vi "Modify Data format to R2 - 複製.vi"(8 "modified error":errorcluster, 10 "original error":errorcluster) -> ()   [LabVIEW 2023]
uses:
  <vilib>/Utility/error.llb/DialogType.ctl
panel:
  in  "Current set number in one current mode":i32=48
  in  "Scan number":i32=10
  out "element":string[](array[string])
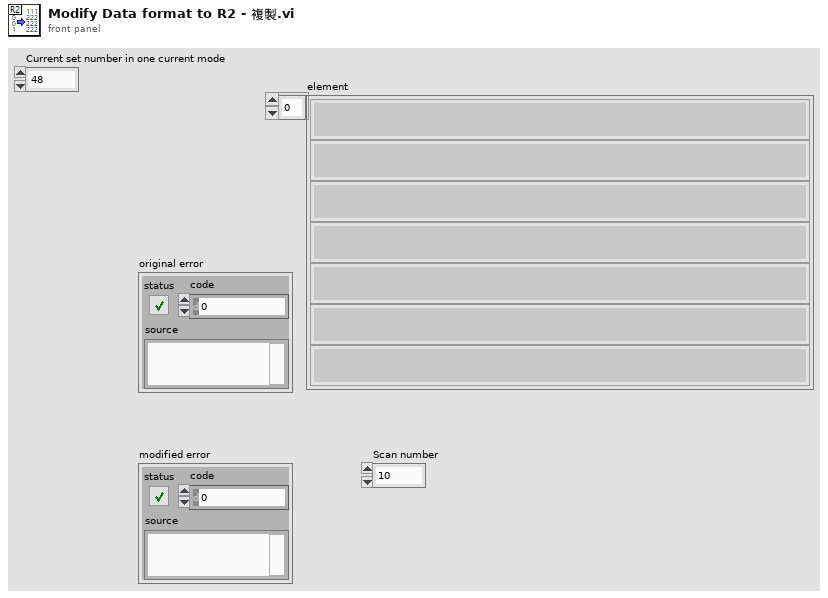
[diagram p1: front panel]
types:
  T1 = enum16{"open", "replace", "create", "open or create", "replace or create", "replace or create with confirmation"}
  T2 = typedef "DialogType.ctl" = u16
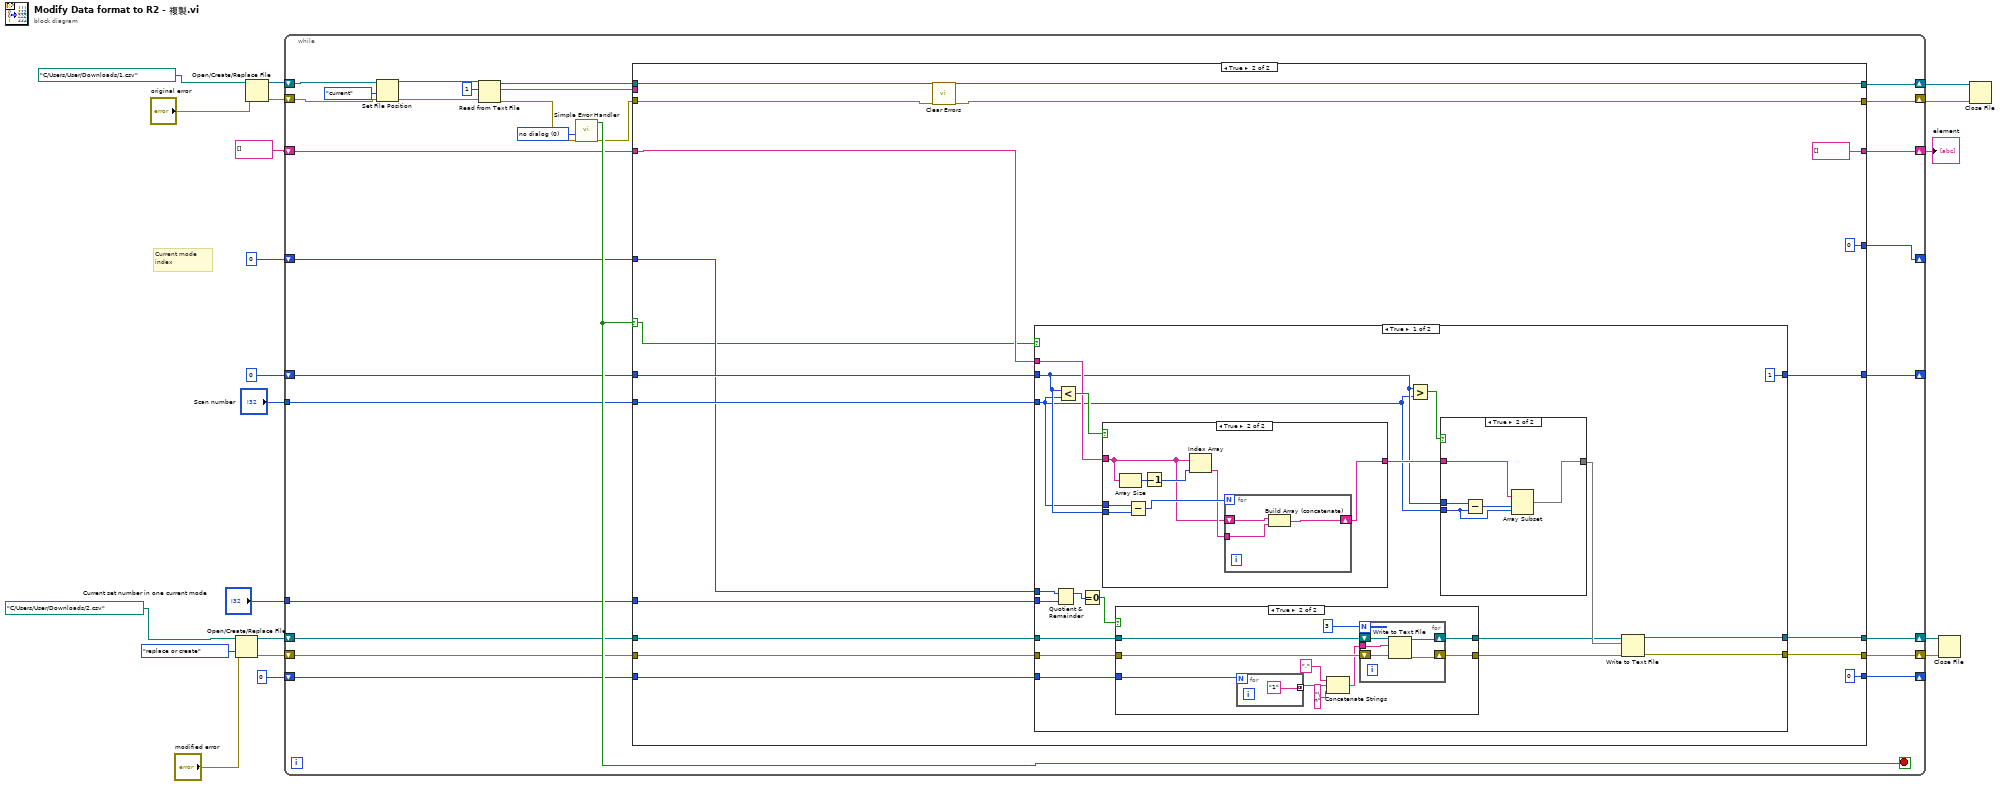
[diagram p0: block diagram]
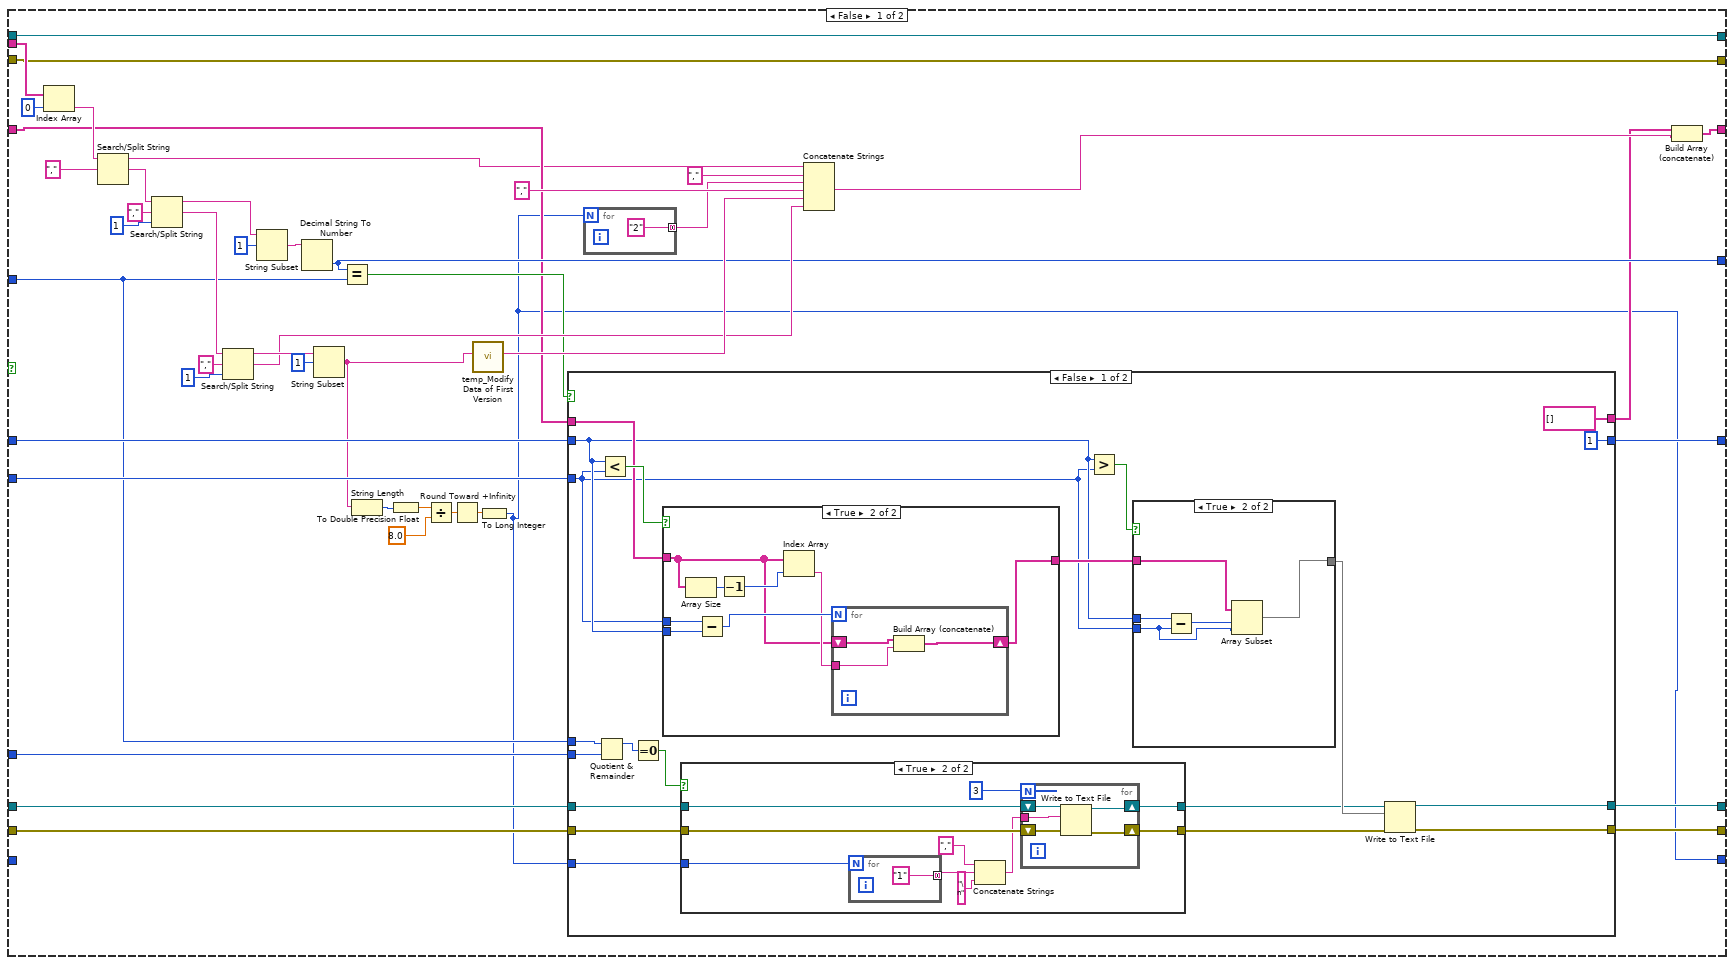
[diagram p2: hidden frame]
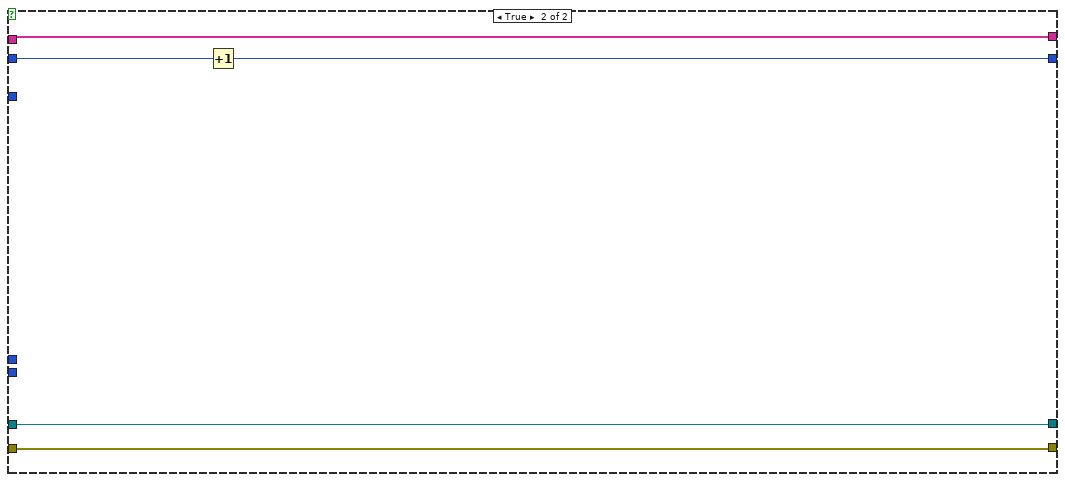
[diagram p6: hidden frame]
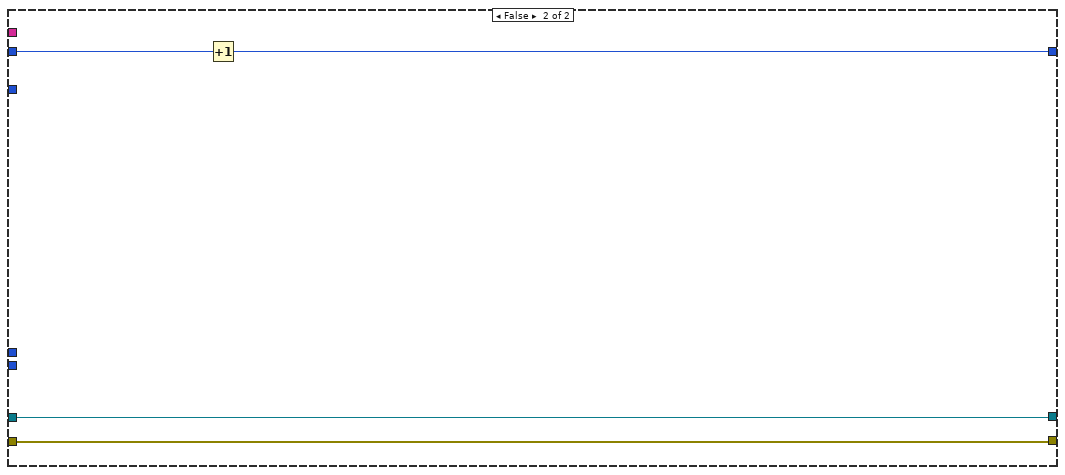
[diagram p10: hidden frame]
diagram:
  # "Current mode\nindex"
  n1 = Open/Create/Replace File(file path (use dialog)=path "C:/Users/User/Downloads/2.csv" ("file path (dialog if empty)"), error in="modified error", operation (0:open)=T1."replace or create") -> (refnum out=w17:refnum<file>, error out=w16:errorcluster)  [unwired: 3 in, 1 out]
  n2 = Open/Create/Replace File(file path (use dialog)=path "C:/Users/User/Downloads/1.csv" ("file path (dialog if empty)"), error in="original error") -> (refnum out=w18:refnum<file>, error out=w19:errorcluster)  [unwired: 4 in, 1 out]
  n3 = while {
    shift-right: [w40] -> w10
    shift-left: w19 -> [w47]
    shift-right: [w39] -> w20
    shift-left: w18 -> [w38]
    shift-right: [w33] -> w12
    shift-left: w17 -> [w35]
    shift-right: [w32] -> w11
    shift-left: w16 -> [w34]
    shift-right: [w21] -> w4
    shift-left: string[] [] ("element") -> [w30]
    shift-right: [w26] -> _
    shift-left: 0 ("number") -> [w29]
    shift-right: [w27] -> _
    shift-left: 0 ("number") -> [w28]
    tunnel: "Scan number" -> [w25]
    tunnel: "Current set number in one current mode" -> [w24]
    shift-right: [w23] -> _
    shift-left: 0 ("32bit integer") -> [w22]
    stop <- w44 stop-if-true
    w45 = T2 0 items=["no dialog", "OK message", "continue or stop message", "OK message + warnings", "continue/stop + warnings"] ("type of dialog (OK msg:1)")
    n4 = Set File Position(refnum=w38, from (0:start)=enum16{"start", "end", "current"}."current", error in=w47) -> (refnum out=w37:refnum<file>, error out=w36:errorcluster)  [unwired: 1 in]
    n5 = Read from Text File(file (use dialog)=w37, count=1, error in=w36) -> (refnum out=w42:refnum<file>, text=w43:string[], error out=w41:errorcluster)  [unwired: 1 in, 1 out]
    n6 = call <vilib>:"Simple Error Handler.vi"("type of dialog (OK msg:1)"=w45, "error in (no error)"=w41) -> ("error?"=w44:bool, "error out"=w31:errorcluster)  [unwired: 3 in, 3 out]
    n7 = case shown="True" w44 {
      selector: w44 -> [_ w160]
      tunnel: w43 -> [w88 _]
      tunnel: w42 -> [w86 w173]
      tunnel: w31 -> [w85 w162]
      tunnel: [w86 w173] -> w39
      tunnel: [w85 w161] -> w40
      tunnel: w35 -> [w65 w168]
      tunnel: w34 -> [w64 w167]
      tunnel: [w63 w166] -> w33
      tunnel: [w62 w165] -> w32
      tunnel: w30 -> [w67 w169]
      tunnel: w29 -> [w61 w164]
      tunnel: w28 -> [w72 w172]
      tunnel: [w71 w171] -> w27
      tunnel: [w70 0] -> w26
      tunnel: w25 -> [w68 w170]
      tunnel: w24 -> [w60 w163]
      tunnel: [w50 0] -> w23
      tunnel: w22 -> [_ w157]
      tunnel: [w49 string[] [] ("element")] -> w21
      frame False {
        n8 = Index Array(array=w88, index=0) -> (element=w84:string)
        n9 = Search/Split String(string=w84, search string/char (-)=",") -> (substring before match=w53:string, match + rest of string=w93:string)  [unwired: 1 in, 1 out]
        n10 = Search/Split String(string=w93, search string/char (-)=",", offset (0)=1) -> (substring before match=w75:string, match + rest of string=w81:string)  [unwired: 1 out]
        n11 = Search/Split String(string=w81, search string/char (-)=",", offset (0)=1) -> (substring before match=w79:string, match + rest of string=w77:string)  [unwired: 1 out]
        n12 = String Subset(string=w75, offset (0)=1) -> (substring=w74:string)  [unwired: 1 in]
        n13 = Decimal String To Number(string=w74) -> (number=w70:i32)  [unwired: 2 in, 1 out]
        n14 = String Subset(string=w79, offset (0)=1) -> (substring=w54:string)  [unwired: 1 in]
        n15 = Equal?(x=w70, y=w61) -> (x = y?=w73:bool)
        n16 = String Length(string=w54) -> (length=w57:i32)
        n17 = To Double Precision Float(number=w57) -> (double precision float=w58:dbl)
        n18 = Divide(x=w58, y=8.0) -> (x/y=w59:dbl)
        n19 = Round Toward +Infinity(x=w59) -> (ceil(x): smallest int >= x=w55:dbl)
        n20 = call "temp_Modify Data of First Version.vi"("string"=w54) -> ("result string 2"=w80:string)  [unwired: 10 in]
        n21 = To Long Integer(number=w55) -> (32bit integer=w50:i32)
        n22 = case shown="False" w73 {
          tunnel: [1 w154] -> w71
          tunnel: w72 -> [w108 w155]
          tunnel: w68 -> [w107 _]
          tunnel: w67 -> [w111 w153]
          tunnel: [string[] [] ("element") w153] -> w66
          tunnel: w65 -> [w99 w152]
          tunnel: w64 -> [w98 w151]
          tunnel: [w105 w152] -> w63
          tunnel: [w104 w151] -> w62
          tunnel: w61 -> [w103 _]
          tunnel: w60 -> [w102 _]
          tunnel: w50 -> [w95 _]
          frame False {
            n23 = Quotient & Remainder(x=w103, y=w102) -> (x-y*floor(x/y)=w101:i32)  [unwired: 1 out]
            n24 = Less?(x=w108, y=w107) -> (x < y?=w112:bool)
            n25 = Equal To 0?(x=w101) -> (x = 0?=w100:bool)
            n26 = case shown="True" w112 {
              tunnel: w111 -> [w139 w141]
              tunnel: w107 -> [_ w145]
              tunnel: w108 -> [_ w144]
              tunnel: [w139 w140] -> w109
              frame False {
              }
              frame True {
                n27 = Array Size(array=w141) -> (size(s)=w147:i32)
                n28 = Subtract(x=w145, y=w144) -> (x-y=w143:i32)
                n29 = Decrement(x=w147) -> (x-1=w146:i32)
                n30 = Index Array(array=w141, index=w146) -> (element=w142:string)
                n31 = for {
                  N: w143 -> [_]
                  tunnel: w142 -> [w148]
                  shift-right: [w149] -> w140
                  shift-left: w141 -> [w150]
                  n32 = Build Array (concatenate)(w150, w148) -> (w149:string[])
                }
              }
            }
            n33 = case shown="True" w100 {
              tunnel: w99 -> [w116 w122]
              tunnel: w98 -> [w115 w121]
              tunnel: [w116 w119] -> w97
              tunnel: [w115 w118] -> w96
              tunnel: w95 -> [_ w117]
              frame False {
              }
              frame True {
                n34 = for {
                  N: w117 -> [_]
                  tunnel: ["1" ("search string/char (-)")] -> w125 mode=concatenating
                }
                n35 = Concatenate Strings("," ("string"), w125, "\n" ("string")) -> (w120:string)
                n36 = for {
                  N: 3 -> [_]
                  shift-right: [w129] -> w119
                  shift-left: w122 -> [w132]
                  tunnel: w120 -> [w130]
                  shift-right: [w128] -> w118
                  shift-left: w121 -> [w131]
                  n37 = Write to Text File(file (use dialog)=w132, text=w130, error in=w131) -> (refnum out=w129:refnum<file>, error out=w128:errorcluster)  [unwired: 1 in, 1 out]
                }
              }
            }
            n38 = Greater?(x=w108, y=w107) -> (0:w110:bool)
            n39 = case shown="True" w110 {
              tunnel: w109 -> [w133 w137]
              tunnel: w108 -> [_ w138]
              tunnel: w107 -> [_ w135]
              tunnel: [w133 w134] -> w106
              frame False {
              }
              frame True {
                n40 = Subtract(x=w138, y=w135) -> (x-y=w136:i32)
                n41 = Array Subset(array=w137, index=w136, length=w135) -> (w134:string[])
              }
            }
            n42 = Write to Text File(file (use dialog)=w97, text=w106, error in=w96) -> (refnum out=w105:refnum<file>, error out=w104:errorcluster)  [unwired: 1 in, 1 out]
          }
          frame True {
            n43 = Increment(x=w155) -> (x+1=w154:i32)
          }
        }
        n44 = for {
          N: w50 -> [_]
          tunnel: ["2" ("search string/char (-)")] -> w51 mode=concatenating
        }
        n45 = Concatenate Strings(w53, "," ("string"), w51, "," ("string"), w80, w77) -> (w69:string)
        n46 = Build Array (concatenate)(w66, w69) -> (w49:string[])
      }
      frame True {
        n47 = call <vilib>:"Clear Errors.vi"("error in (no error)"=w162) -> ("error out"=w161:errorcluster)  [unwired: 5 in, 1 out]
        n48 = case shown="True" w160 {
          tunnel: [1 w231] -> w171
          tunnel: w172 -> [w187 w232]
          tunnel: w170 -> [w186 _]
          tunnel: w169 -> [w190 _]
          tunnel: w168 -> [w178 w230]
          tunnel: w167 -> [w177 w229]
          tunnel: [w184 w230] -> w166
          tunnel: [w183 w229] -> w165
          tunnel: w164 -> [w182 _]
          tunnel: w163 -> [w181 _]
          tunnel: w157 -> [w174 _]
          frame True {
            n49 = Quotient & Remainder(x=w182, y=w181) -> (x-y*floor(x/y)=w180:i32)  [unwired: 1 out]
            n50 = Less?(x=w187, y=w186) -> (x < y?=w191:bool)
            n51 = Equal To 0?(x=w180) -> (x = 0?=w179:bool)
            n52 = case shown="True" w191 {
              tunnel: w190 -> [w217 w219]
              tunnel: w186 -> [_ w223]
              tunnel: w187 -> [_ w222]
              tunnel: [w217 w218] -> w188
              frame False {
              }
              frame True {
                n53 = Array Size(array=w219) -> (size(s)=w225:i32)
                n54 = Subtract(x=w223, y=w222) -> (x-y=w221:i32)
                n55 = Decrement(x=w225) -> (x-1=w224:i32)
                n56 = Index Array(array=w219, index=w224) -> (element=w220:string)
                n57 = for {
                  N: w221 -> [_]
                  tunnel: w220 -> [w226]
                  shift-right: [w227] -> w218
                  shift-left: w219 -> [w228]
                  n58 = Build Array (concatenate)(w228, w226) -> (w227:string[])
                }
              }
            }
            n59 = case shown="True" w179 {
              tunnel: w178 -> [w194 w200]
              tunnel: w177 -> [w193 w199]
              tunnel: [w194 w197] -> w176
              tunnel: [w193 w196] -> w175
              tunnel: w174 -> [_ w195]
              frame False {
              }
              frame True {
                n60 = for {
                  N: w195 -> [_]
                  tunnel: ["1" ("search string/char (-)")] -> w203 mode=concatenating
                }
                n61 = Concatenate Strings("," ("string"), w203, "\n" ("string")) -> (w198:string)
                n62 = for {
                  N: 3 -> [_]
                  shift-right: [w207] -> w197
                  shift-left: w200 -> [w210]
                  tunnel: w198 -> [w208]
                  shift-right: [w206] -> w196
                  shift-left: w199 -> [w209]
                  n63 = Write to Text File(file (use dialog)=w210, text=w208, error in=w209) -> (refnum out=w207:refnum<file>, error out=w206:errorcluster)  [unwired: 1 in, 1 out]
                }
              }
            }
            n64 = Greater?(x=w187, y=w186) -> (0:w189:bool)
            n65 = case shown="True" w189 {
              tunnel: w188 -> [w211 w215]
              tunnel: w187 -> [_ w216]
              tunnel: w186 -> [_ w213]
              tunnel: [w211 w212] -> w185
              frame False {
              }
              frame True {
                n66 = Subtract(x=w216, y=w213) -> (x-y=w214:i32)
                n67 = Array Subset(array=w215, index=w214, length=w213) -> (w212:string[])
              }
            }
            n68 = Write to Text File(file (use dialog)=w176, text=w185, error in=w175) -> (refnum out=w184:refnum<file>, error out=w183:errorcluster)  [unwired: 1 in, 1 out]
          }
          frame False {
            n69 = Increment(x=w232) -> (x+1=w231:i32)
          }
        }
      }
    }
  }
  "element" <- w4
  n70 = Close File(refnum=w12, error in=w11) -> ()  [unwired: 2 out]
  n71 = Close File(refnum=w20, error in=w10) -> ()  [unwired: 2 out]
